vi "camera_release_configuration.vi"(2 "error in":errorcluster, 3 "Session In":T1, 4 "Ereignisregistrierung (Referenz) 2":refnum<event-registration>) -> (0 "error out":errorcluster, 1 "Session Out":T1)   [LabVIEW 2009]
uses:
  <vilib>/userDefined/High Color/IMAQdx.ctl
  <vilib>/vision/driver/NI_Vision_Acquisition_Software.lvlib
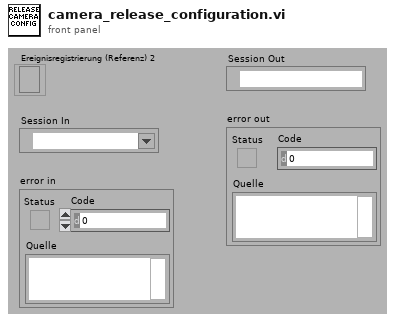
[diagram p1: front panel]
types:
  T1 = typedef "IMAQdx.ctl" = refnum<k21>
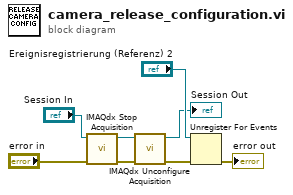
[diagram p0: block diagram]
diagram:
  n1 = call <vilib>:"IMAQdx Stop Acquisition.vi"("error in"="error in", "Session In"="Session In") -> ("error out"=w2:errorcluster, "Session Out"=w3:T1)  [unwired: 8 in]
  n2 = call <vilib>:"IMAQdx Unconfigure Acquisition.vi"("error in"=w2, "Session In"=w3) -> ("error out"=w4:errorcluster, "Session Out"=→"Session Out":T1)  [unwired: 8 in]
  n3 = Unregister For Events(event registration refnum="Ereignisregistrierung (Referenz) 2", error in=w4) -> (error out=→"error out":errorcluster)
